vi "Get File Version Info.vi"(2 "error in (no error)":errorcluster, 3 "File path":path) -> (0 "error out":errorcluster, 1 "File Version":string)   [LabVIEW 2018, in "Tracker.lvlib"]
uses:
  Tracker.lvlib
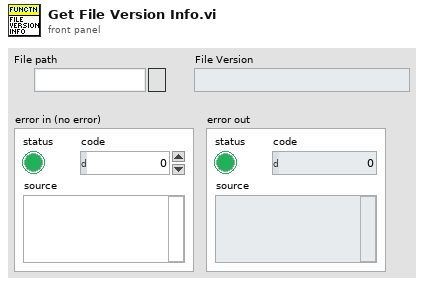
[diagram p1: front panel]
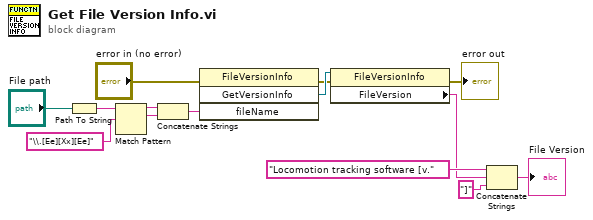
[diagram p0: block diagram]
diagram:
  n1 = Path To String(path="File path") -> (string=w9:string)
  n2 = Match Pattern(string=w9, regular expression="\\.[Ee][Xx][Ee]") -> (before substring=w11:string, match substring=w12:string)  [unwired: 1 in, 2 out]
  n3 = Concatenate Strings(w11, w12) -> (w10:string)
  n4 = invoke class="FileVersionInfo" method="GetVersionInfo"(error in="error in (no error)", "fileName"=w10) -> (error out=w6:errorcluster, "GetVersionInfo"=w14:refnum<k24>)  [unwired: 2 in, 2 out]
  n5 = property class="FileVersionInfo"(reference=w14, error in=w6) -> (error out=→"error out":errorcluster, "FileVersion"=w2:string)  [unwired: 1 out]
  n6 = Concatenate Strings("Locomotion tracking software [v." ("string"), w2, "]" ("string")) -> (→"File Version":string)
